vi "TR_Calc_phi_theta_etc_2_(offline).vi"(0 "Input data cluster":T2, 1 "SB size":u8, 5 "Twisted neck":bool, 7 "Bridge swap":bool, 9 "Use alternative magnets orientation":bool, 11 "Error In":errorcluster) -> (4 "Animal coordinates cluster":T1, 15 "Error out":errorcluster)   [LabVIEW 2018, in "Tracks Repair.lvlib"]
uses:
  Tracks Repair.lvlib
  SubVi's/Controls/CTL_Cage_Coords_(arrays).ctl
  SubVi's/Controls/CTL_Animal_Coordinates_and_Speed_(arr).ctl
  SubVi's/Controls/CTL_Animal_Coordinates_and_Speed.ctl
  Tracker.lvlib
  <vilib>/ptbypt/NI_PtbyPt.lvlib
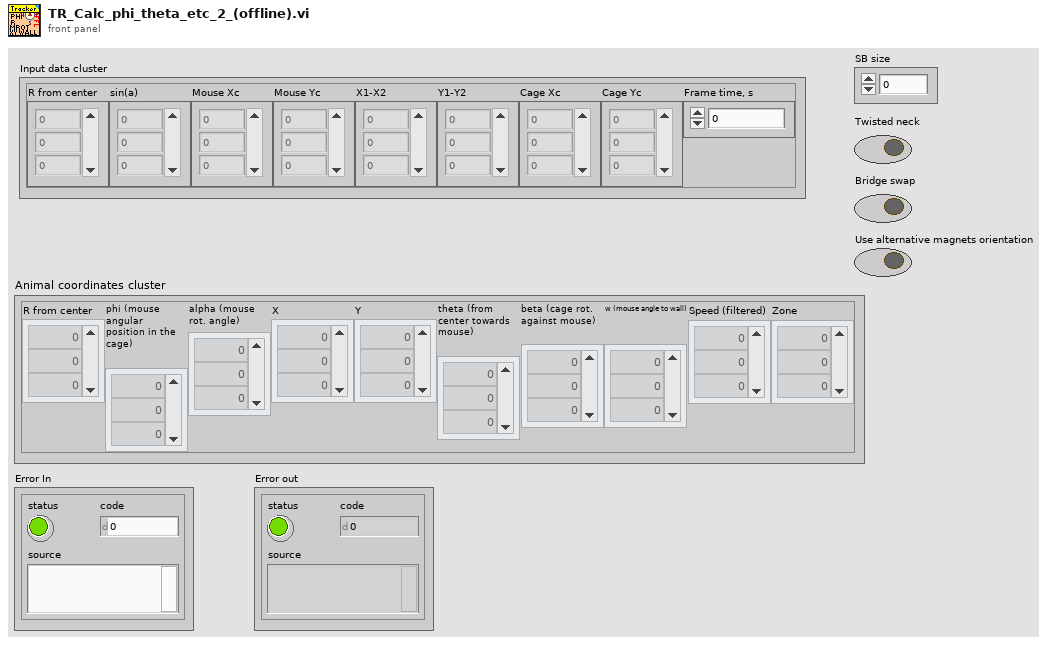
[diagram p1: front panel]
types:
  T1 = typedef "Tracker.lvlib/CTL_Animal_Coordinates_and_Speed_(arr).ctl" = cluster{"R from center":dbl[], "phi (mouse angular position in the cage)":dbl[], "alpha (mouse rot. angle)":dbl[], "X":dbl[], "Y":dbl[], "theta (from center towards mouse)":dbl[], "beta (cage rot. against mouse)":dbl[], "w (mouse angle to wall)":dbl[], "Speed (filtered)":dbl[], "Zone":i8[]}
  T2 = typedef "Tracker.lvlib/CTL_Cage_Coords_(arrays).ctl" = cluster{"R from center":dbl[], "sin(a)":dbl[], "Mouse Xc":dbl[], "Mouse Yc":dbl[], "X1-X2":dbl[], "Y1-Y2":dbl[], "Cage Xc":dbl[], "Cage Yc":dbl[], "Frame time, s":dbl}
  T3 = typedef "Tracker.lvlib/CTL_Animal_Coordinates_and_Speed.ctl" = cluster{"R from center":dbl, "phi (mouse angular position in the cage)":dbl, "alpha (mouse rot. angle)":dbl, "X":dbl, "Y":dbl, "theta (from center towards mouse)":dbl, "beta (cage rot. against mouse)":dbl, "w (mouse angle to wall)":dbl, "Speed (filtered)":dbl}
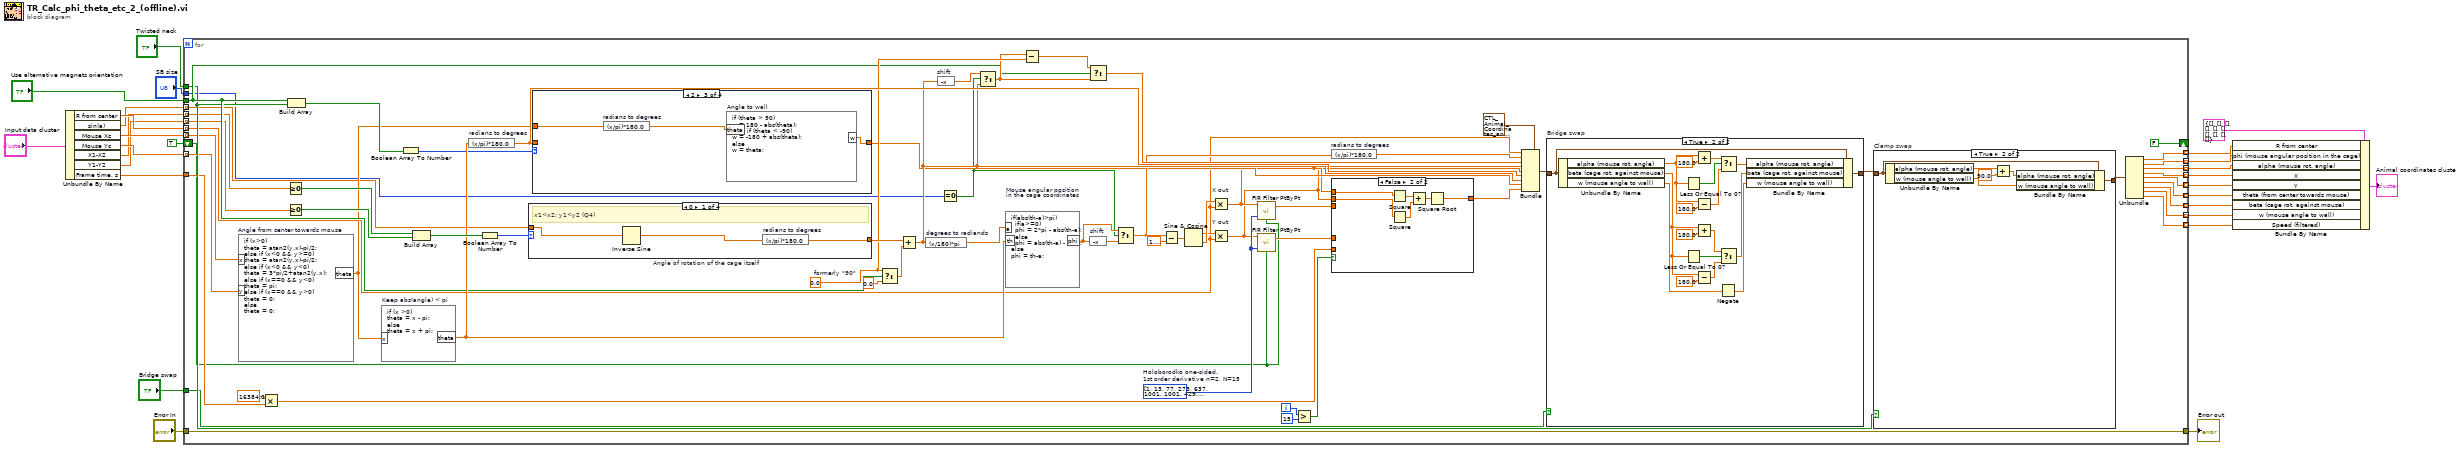
[diagram p0: block diagram]
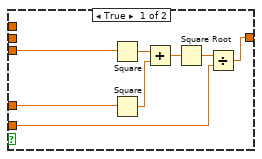
[diagram p2: hidden frame]
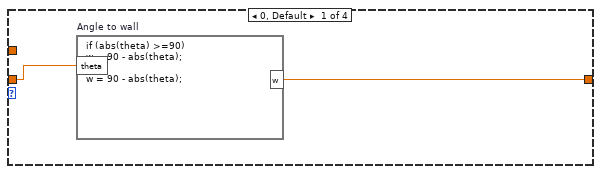
[diagram p4: hidden frame]
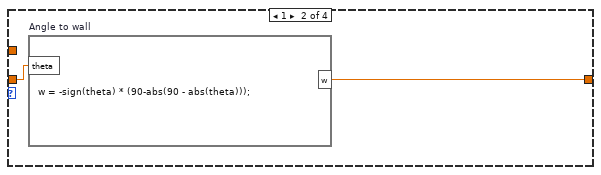
[diagram p5: hidden frame]
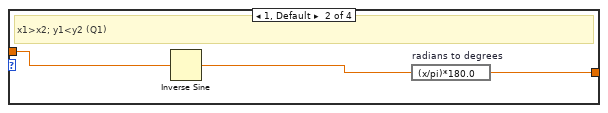
[diagram p8: hidden frame]
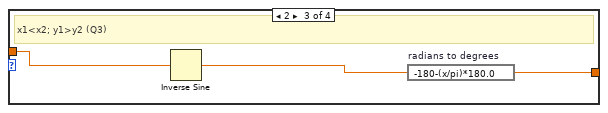
[diagram p9: hidden frame]
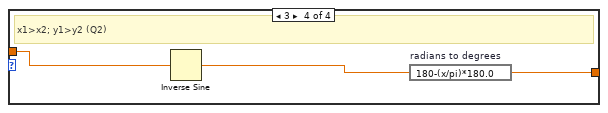
[diagram p10: hidden frame]
diagram:
  n1 = Unbundle By Name("Input data cluster") -> ("R from center"=w22:dbl[], "sin(a)"=w21:dbl[], "Mouse Xc"=w20:dbl[], "Mouse Yc"=w19:dbl[], "X1-X2"=w18:dbl[], "Y1-Y2"=w17:dbl[], "Frame time, s"=w16:dbl)
  n2 = for {
    tunnel: "Use alternative magnets orientation" -> [w66]
    tunnel: "Twisted neck" -> [w65]
    tunnel: "SB size" -> [w61]
    tunnel: "Bridge swap" -> [w53]
    tunnel: w22 -> [w52] mode=indexing
    tunnel: w21 -> [w51] mode=indexing
    tunnel: w20 -> [w50] mode=indexing
    tunnel: w19 -> [w49] mode=indexing
    tunnel: w18 -> [w48] mode=indexing
    tunnel: w17 -> [w47] mode=indexing
    tunnel: w16 -> [w46]
    tunnel: [w44] -> w13 mode=indexing
    tunnel: [w43] -> w12 mode=indexing
    tunnel: [w42] -> w11 mode=indexing
    tunnel: [w41] -> w10 mode=indexing
    tunnel: [w40] -> w9 mode=indexing
    tunnel: [w39] -> w8 mode=indexing
    tunnel: [w38] -> w7 mode=indexing
    tunnel: [w37] -> w6 mode=indexing
    tunnel: [w36] -> w5 mode=indexing
    tunnel: "Error In" -> [w35]
    tunnel: [w35] -> w3
    shift-right: [FALSE] -> _
    shift-left: TRUE -> [w34]
    i -> [w31]
    w59 = i32[] [1, 13, 77, 273, 637, 1001, 1001, 429, -429, -1001, -1001, -637, -273, -77, -13, -1]  # Holoborodko one-sided, 1st order derivative n=2, N=15
    w76 = 0.0  # formerly "90"
    n3 = formula code="if (x>0)\ntheta = atan2(y,x)-pi/2;\nelse if (x<0 && y>=0)\ntheta = atan2(y,x)-pi/2;\nelse if (x<0 && y<0)\ntheta = 3*pi/2+atan2(y,x);\nelse if (x==0 && y<0)\ntheta = pi;\nelse if (x==0 && y>0)\ntheta = 0;\nelse\ntheta = 0;" "Angle from center towards mouse"("x"=w50, "y"=w49) -> ("theta"=w62:dbl)
    n4 = Multiply(x=16384.0 ("y"), y=w46) -> (x*y=w54:dbl)
    n5 = Greater Or Equal To 0?(x=w48) -> (x >= 0?=w93:bool)
    n6 = Greater Or Equal To 0?(x=w47) -> (x >= 0?=w92:bool)
    n7 = Build Array(w66, w65) -> (w64:bool[])
    n8 = formula code="if (x >0)\ntheta = x - pi;\nelse\ntheta = x + pi;" "Keep abs(angle) < pi"("x"=w62) -> ("theta"=w87:dbl)
    n9 = Boolean Array To Number(Boolean array=w64) -> (number=w63:u32)
    n10 = Build Array(w93, w92) -> (w91:bool[])
    n11 = expression code="(x/pi)*180.0" "radians to degrees"(w87) -> (w83:dbl)
    n12 = Boolean Array To Number(Boolean array=w91) -> (number=w90:u32)
    n13 = case "Angle of rotation of the cage itself" shown="0" w90 {
      tunnel: w51 -> [w143 w146 w149 w152]
      tunnel: [w142 w145 w148 w151] -> w79
      frame 0 {
        # "x1<x2; y1<y2 (Q4)"
        n14 = Inverse Sine(1:w143) -> (0:w144:dbl)
        n15 = expression code="(x/pi)*180.0" "radians to degrees"(w144) -> (w142:dbl)
      }
      frame 1, Default {
        # "x1>x2; y1<y2 (Q1)"
        n16 = Inverse Sine(1:w146) -> (0:w147:dbl)
        n17 = expression code="(x/pi)*180.0" "radians to degrees"(w147) -> (w145:dbl)
      }
      frame 2 {
        # "x1<x2; y1>y2 (Q3)"
        n18 = Inverse Sine(1:w149) -> (0:w150:dbl)
        n19 = expression code="-180-(x/pi)*180.0" "radians to degrees"(w150) -> (w148:dbl)
      }
      frame 3 {
        # "x1>x2; y1>y2 (Q2)"
        n20 = Inverse Sine(1:w152) -> (0:w153:dbl)
        n21 = expression code="180-(x/pi)*180.0" "radians to degrees"(w153) -> (w151:dbl)
      }
    }
    n22 = case shown="2" w63 {
      tunnel: w83 -> [w116 w118 _ w122]
      tunnel: [w115 w117 w121 w122] -> w67
      tunnel: w62 -> [_ _ w120 _]
      frame 0, Default {
        n23 = formula code="if (abs(theta) >=90)\nw = 90 - abs(theta);\nelse\nw = 90 - abs(theta);" "Angle to wall"("theta"=w116) -> ("w"=w115:dbl)
      }
      frame 1 {
        n24 = formula code="w = -sign(theta) * (90-abs(90 - abs(theta)));" "Angle to wall"("theta"=w118) -> ("w"=w117:dbl)
      }
      frame 2 {
        n25 = expression code="(x/pi)*180.0" "radians to degrees"(w120) -> (w119:dbl)
        n26 = formula code="if (theta > 90)\nw = 180 - abs(theta);\nelse if (theta < -90)\nw = -180 + abs(theta);\nelse\nw = theta;" "Angle to wall"("theta"=w119) -> ("w"=w121:dbl)
      }
      frame 3 {
      }
    }
    n27 = Select(t=w76, s=w66, f=0.0) -> (s? t:f=w75:dbl)
    n28 = Add(x=w79, y=w75) -> (x+y=w73:dbl)
    n29 = expression code="(x/180)*pi" "degrees to radiands"(w73) -> (w86:dbl)
    n30 = expression code="-x" "shift"(w73) -> (w72:dbl)
    n31 = Equal To 0?(x=w61) -> (x = 0?=w60:bool)
    n32 = Select(t=w72, s=w60, f=w73) -> (s? t:f=w74:dbl)
    n33 = formula code="if(abs(th-a)>pi)\n  if(a>=0)\n  phi = 2*pi - abs(th-a);\n  else\n  phi = abs(th-a) - 2*pi;\nelse\nphi = th-a;" "Mouse angular position in the cage coordinates"("th"=w87, "a"=w86) -> ("phi"=w70:dbl)
    n34 = Subtract(x=w74, y=w76) -> (x-y=w77:dbl)
    n35 = Select(t=w77, s=w66, f=w74) -> (s? t:f=w78:dbl)
    n36 = expression code="-x" "shift"(w70) -> (w69:dbl)
    n37 = Select(t=w70, s=w60, f=w69) -> (s? t:f=w71:dbl)
    n38 = Subtract(x=w71, y=1.5707963267948966) -> (x-y=w85:dbl)
    n39 = Sine & Cosine(0:w85) -> (1:w88:dbl, 2:w89:dbl)
    n40 = Multiply "X out"(x=w89, y=w52) -> (x*y=w28:dbl)
    n41 = Multiply "Y out"(x=w88, y=w52) -> (x*y=w27:dbl)
    n42 = call <vilib>:"FIR Filter PtByPt.vi"("initialize"=w34, "Forward Coefficients"=w59, "x"=w28) -> ("Filtered x"=w58:dbl)  [unwired: 1 in, 1 out]
    n43 = call <vilib>:"FIR Filter PtByPt.vi"("initialize"=w34, "Forward Coefficients"=w59, "x"=w27) -> ("Filtered x"=w57:dbl)  [unwired: 1 in, 1 out]
    n44 = Greater?(x=w31, y=15) -> (0:w29:bool)
    n45 = expression code="(x/pi)*180.0" "radians to degrees"(w71) -> (w82:dbl)
    n46 = case shown="False" w29 {
      tunnel: w58 -> [w101 _]
      tunnel: w57 -> [w100 _]
      tunnel: [w96 w104] -> w56
      tunnel: w54 -> [w94 _]
      tunnel: w28 -> [_ w103]
      tunnel: w27 -> [_ w102]
      frame True {
        n47 = Square(x=w101) -> (x^2=w99:dbl)
        n48 = Square(x=w100) -> (x^2=w98:dbl)
        n49 = Add(x=w99, y=w98) -> (x+y=w97:dbl)
        n50 = Square Root(x=w97) -> (sqrt(x)=w95:dbl)
        n51 = Divide(x=w95, y=w94) -> (x/y=w96:dbl)
      }
      frame False {
        n52 = Square(x=w103) -> (x^2=w107:dbl)
        n53 = Square(x=w102) -> (x^2=w106:dbl)
        n54 = Add(x=w107, y=w106) -> (x+y=w105:dbl)
        n55 = Square Root(x=w105) -> (sqrt(x)=w104:dbl)
      }
    }
    n56 = Bundle(cluster=T3 {"R from center"=0.0, "phi (mouse angular position in the cage)"=0.0, "alpha (mouse rot. angle)"=0.0, "X"=0.0, "Y"=0.0, "theta (from center towards mouse)"=0.0, "beta (cage rot. against mouse)"=0.0, "w (mouse angle to wall)"=0.0, "Speed (filtered)"=0.0} ("Animal coordinates and speed"), "R from center"=w52, "phi (mouse angular position in the cage)"=w82, "alpha (mouse rot. angle)"=w78, "X"=w28, "Y"=w27, "theta (from center towards mouse)"=w83, "beta (cage rot. against mouse)"=w73, "w (mouse angle to wall)"=w67, "Speed (filtered)"=w56) -> (w81:T3)
    n57 = case "Bridge swap" shown="True" w53 {
      tunnel: [w123 w135] -> w68
      tunnel: w81 -> [w123 w136]
      frame False {
      }
      frame True {
        n58 = Unbundle By Name(w136) -> ("alpha (mouse rot. angle)"=w134:dbl, "beta (cage rot. against mouse)"=w127:dbl, "w (mouse angle to wall)"=w125:dbl)
        n59 = Less Or Equal To 0?(x=w134) -> (x <= 0?=w141:bool)
        n60 = Less Or Equal To 0?(x=w127) -> (x <= 0?=w128:bool)
        n61 = Add(x=w134, y=sgl 180.0) -> (x+y=w138:dbl)
        n62 = Subtract(x=w134, y=sgl 180.0) -> (x-y=w140:dbl)
        n63 = Add(x=w127, y=sgl 180.0) -> (x+y=w131:dbl)
        n64 = Subtract(x=w127, y=sgl 180.0) -> (x-y=w129:dbl)
        n65 = Negate(x=w125) -> (-x=w124:dbl)
        n66 = Select(t=w138, s=w141, f=w140) -> (s? t:f=w133:dbl)
        n67 = Select(t=w131, s=w128, f=w129) -> (s? t:f=w126:dbl)
        n68 = Bundle By Name(cluster=w136, "alpha (mouse rot. angle)"=w133, "beta (cage rot. against mouse)"=w126, "w (mouse angle to wall)"=w124) -> (w135:T3)
      }
    }
    n69 = case "Clamp swap" shown="True" w65 {
      tunnel: [w108 w112] -> w45
      tunnel: w68 -> [w108 w113]
      frame False {
      }
      frame True {
        n70 = Unbundle By Name(w113) -> ("alpha (mouse rot. angle)"=w111:dbl, "w (mouse angle to wall)"=w110:dbl)
        n71 = Add(x=w111, y=sgl 90.0) -> (x+y=w109:dbl)
        n72 = Bundle By Name(cluster=w113, "alpha (mouse rot. angle)"=w109, "w (mouse angle to wall)"=w110) -> (w112:T3)
      }
    }
    n73 = Unbundle(w45) -> ("R from center"=w44:dbl, "phi (mouse angular position in the cage)"=w43:dbl, "alpha (mouse rot. angle)"=w42:dbl, "X"=w41:dbl, "Y"=w40:dbl, "theta (from center towards mouse)"=w39:dbl, "beta (cage rot. against mouse)"=w38:dbl, "w (mouse angle to wall)"=w37:dbl, "Speed (filtered)"=w36:dbl)
  }
  "Error out" <- w3
  n74 = Bundle By Name(cluster=T1 {"R from center"=[], "phi (mouse angular position in the cage)"=[], "alpha (mouse rot. angle)"=[], "X"=[], "Y"=[], "theta (from center towards mouse)"=[], "beta (cage rot. against mouse)"=[], "w (mouse angle to wall)"=[], "Speed (filtered)"=[], "Zone"=[]} ("Animal coordinates and speed"), "R from center"=w13, "phi (mouse angular position in the cage)"=w12, "alpha (mouse rot. angle)"=w11, "X"=w10, "Y"=w9, "theta (from center towards mouse)"=w8, "beta (cage rot. against mouse)"=w7, "w (mouse angle to wall)"=w6, "Speed (filtered)"=w5) -> (→"Animal coordinates cluster":T1)
